vi "InitFromXML.vi"(8 "error in (no error)":errorcluster, 10 "XML":string, 11 "SystemExec in":refnum<class "SystemExec.lvclass">) -> (0 "error out":errorcluster, 3 "SystemExec out":refnum<class "SystemExec.lvclass">)   [LabVIEW 2009, in "NavScreen.lvlib" / "SystemExec.lvclass"]
uses:
  SystemExec.lvclass
  ClickableText/ClickableText.lvclass
  SystemExec.lvclass/SystemExec.ctl
  NavScreen.lvlib
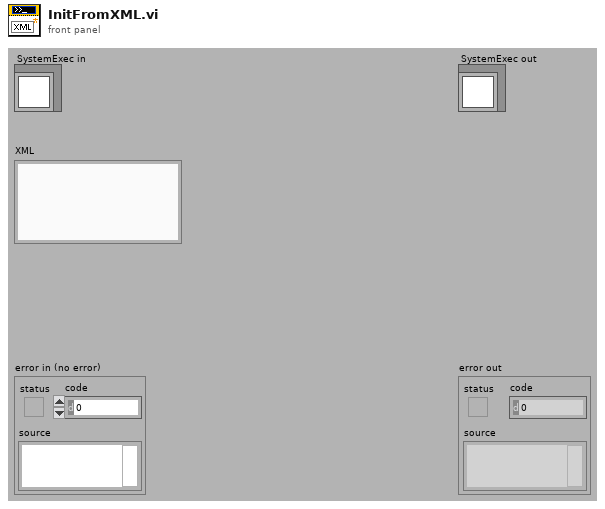
[diagram p1: front panel]
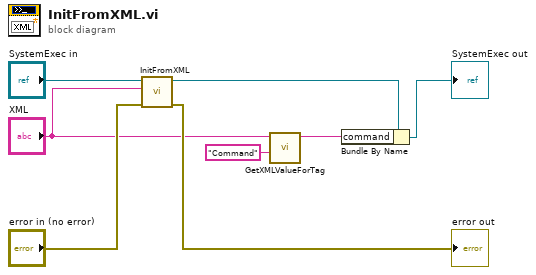
[diagram p0: block diagram]
diagram:
  n1 = call-parent "InitFromXML.vi"("error in (no error)"="error in (no error)", "XML"="XML", "ClickableText in"="SystemExec in") -> ("error out"=→"error out":errorcluster, "ClickableText out"=w3:refnum<class "SystemExec.lvclass">)  [unwired: 7 in]
  n2 = call "GetXMLValueForTag.vi"("tag"="Command", "XML"="XML") -> ("value"=w2:string)  [unwired: 8 in, 1 out]
  n3 = Bundle By Name(cluster=w3, "command"=w2) -> (→"SystemExec out":refnum<class "SystemExec.lvclass">)
